vi "Read VISA.vi"(8 "error in (no error)":errorcluster, 11 "ElectrometerConfiguration in":refnum<class "ElectrometerCOMConfiguration.lvclass">) -> (0 "error out":errorcluster, 2 "VISA":refnum<visa-resource-name>, 3 "ElectrometerConfiguration out":refnum<class "ElectrometerCOMConfiguration.lvclass">)   [LabVIEW 2016, in "ElectrometerCOMConfiguration.lvclass"]
uses:
  ElectrometerCOMConfiguration.lvclass
  ElectrometerCOMConfiguration.lvclass/ElectrometerCOMConfiguration.ctl
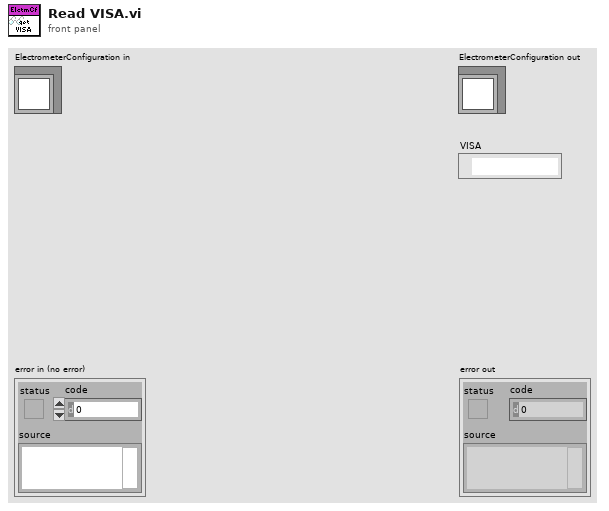
[diagram p1: front panel]
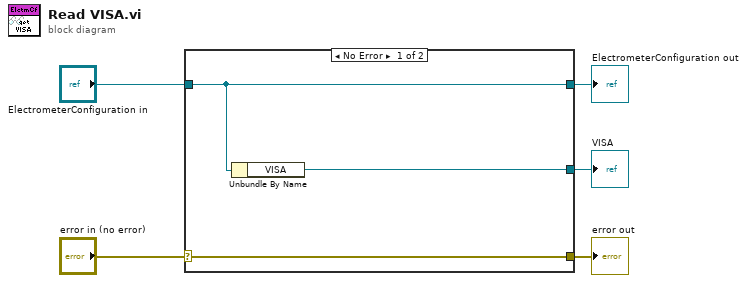
[diagram p0: block diagram]
diagram:
  n1 = case shown="No Error" "error in (no error)" {
    selector: "error in (no error)" -> [w8 w9]
    tunnel: [w8 w9] -> w4
    tunnel: [w7 w10] -> w2
    tunnel: "ElectrometerConfiguration in" -> [w7 w10]
    tunnel: [w6 _] -> w1
    frame No Error {
      n2 = Unbundle By Name(w7) -> ("VISA"=w6:refnum<visa-resource-name>)
    }
    frame Error {
    }
  }
  "error out" <- w4
  "ElectrometerConfiguration out" <- w2
  "VISA" <- w1
